vi "p1.vi"() -> ()   [LabVIEW 2025, in "d4.lvlib"]
uses:
  d4.lvlib
  AOC/AOC.lvlib
  <userlib>/_OpenG.lib/string/string.llb/openg_string.lvlib
panel:
  in  "Example":string="..@@.@@@@.\n@@@.@.@.@@\n@@@@@.@.@@\n@.@@@@..@.\n@@.@@@@.@@\n.@@@@@@@.@\n.@.@.@.@@@\n@.@@@.@@@@\n.@@@@@@@@.\n@.@.@@@.@."
  in  "Example":bool
  out "Answer":i64=605
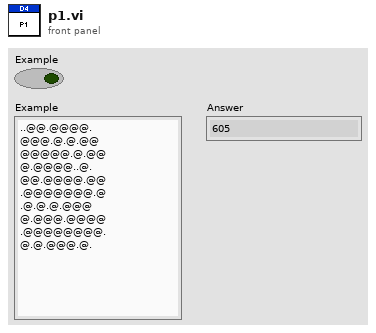
[diagram p1: front panel]
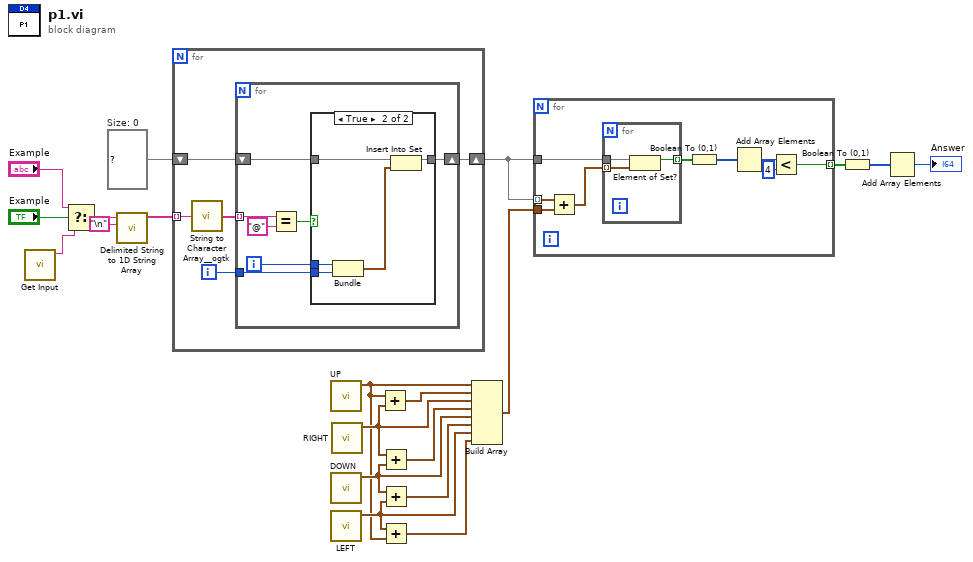
[diagram p0: block diagram]
diagram:
  w15 = set{cluster{i32, i32}} {}  # Size: 0
  n1 = call "Get Input.vi"() -> ("Input"=w20:string)  [unwired: 11 in]
  n2 = Select(t="Example", s="Example", f=w20) -> (s? t:f=w17:string)
  n3 = call <vilib>:"Delimited String to 1D String Array.vi"("delimiter"="\n", "delimited string"=w17) -> ("string array"=w16:string[])  [unwired: 9 in]
  n4 = for {
    tunnel: w16 -> [w25] mode=indexing
    shift-right: [w21] -> w14
    shift-left: w15 -> [w22]
    i -> [w23]
    n5 = call <userlib>:"String to Character Array__ogtk.vi"("Input String"=w25) -> ("Character Array"=w24:string[])
    n6 = for {
      tunnel: w24 -> [w32] mode=indexing
      tunnel: w23 -> [w29]
      shift-right: [w26] -> w21
      shift-left: w22 -> [w27]
      i -> [w28]
      n7 = Equal?(x=w32, y="@") -> (x = y?=w30:bool)
      n8 = case shown="True" w30 {
        tunnel: w29 -> [_ w38]
        tunnel: w28 -> [_ w37]
        tunnel: w27 -> [w33 w36]
        tunnel: [w33 w34] -> w26
        frame False {
        }
        frame True {
          n9 = Bundle(w37, w38) -> (w35:cluster{i32, i32})  [unwired: 1 in]
          n10 = Insert Into Set(10:w35, 11:w36) -> (3:w34:set{cluster{i32, i32}})  [unwired: 1 out]
        }
      }
    }
  }
  n11 = call "UP.vi"() -> ("UP"=w7:cluster{"x":i16, "y":i16})  [unwired: 11 in]
  n12 = call "DOWN.vi"() -> ("DOWN"=w9:cluster{"x":i16, "y":i16})  [unwired: 11 in]
  n13 = call "LEFT.vi"() -> ("LEFT"=w8:cluster{"x":i16, "y":i16})  [unwired: 11 in]
  n14 = call "RIGHT.vi"() -> ("RIGHT"=w12:cluster{"x":i16, "y":i16})  [unwired: 11 in]
  n15 = Add(x=w7, y=w12) -> (x+y=w13:cluster{"x":i16, "y":i16})
  n16 = Add(x=w12, y=w9) -> (x+y=w11:cluster{"x":i16, "y":i16})
  n17 = Add(x=w9, y=w8) -> (x+y=w10:cluster{"x":i16, "y":i16})
  n18 = Add(x=w8, y=w7) -> (x+y=w6:cluster{"x":i16, "y":i16})
  n19 = Build Array(w7, w13, w12, w11, w9, w10, w8, w6) -> (w5:cluster{"x":i16, "y":i16}[])
  n20 = for {
    tunnel: w14 -> [w47] mode=indexing
    tunnel: w14 -> [w45]
    tunnel: w5 -> [w46]
    tunnel: [w39] -> w3 mode=indexing
    n21 = Add(x=w47, y=w46) -> (x+y=w44:cluster{i32, i32}[])
    n22 = for {
      tunnel: w45 -> [w50]
      tunnel: w44 -> [w49] mode=indexing
      tunnel: [w48] -> w43 mode=indexing
      n23 = Element of Set?(10:w49, 11:w50) -> (3:w48:bool)
    }
    n24 = Boolean To (0,1)(Boolean=w43) -> (0, 1=w42:i16[])
    n25 = Add Array Elements(numeric array=w42) -> (sum=w41:i16)
    n26 = Less?(x=w41, y=i16 4) -> (x < y?=w39:bool)
  }
  n27 = Boolean To (0,1)(Boolean=w3) -> (0, 1=w4:i16[])
  n28 = Add Array Elements(numeric array=w4) -> (sum=→"Answer":i16)
